vi "Set Output Values.vi"(8 "Error In":errorcluster, 9 "Start Index":i32, 10 "Values":dbl[](array[numeric]), 11 "BNT_ULx-MCSV in":refnum<class "BNT_ULx-MCSV.lvclass">) -> (0 "Error Out":errorcluster, 3 "BNT_ULx-MCSV out":refnum<class "BNT_ULx-MCSV.lvclass">)   [LabVIEW 2020, in "BNT_ULx.lvlib" / "BNT_ULx-MCSV.lvclass"]
doc: "Write voltage values to DAQmx device and publish.\n\nTimeout is set to constant 1s."
uses:
  BNT_ULx-MCSV.lvclass
  BNT_ULx-MCSV.lvclass/BNT_ULx-MCSV.ctl
  <vilib>/ULx/Write.llb/ULx Write (Analog 1D DBL NChan 1Samp).vi
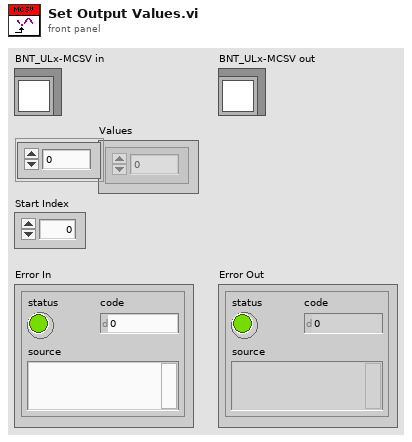
[diagram p1: front panel]
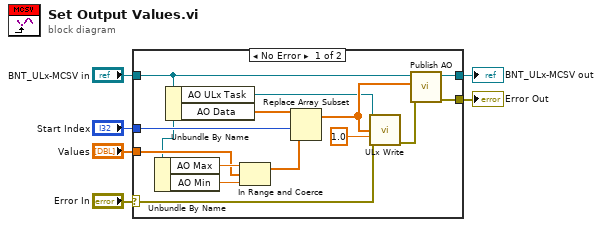
[diagram p0: block diagram]
diagram:
  n1 = case shown="No Error" "Error In" {
    selector: "Error In" -> [w10 w22]
    tunnel: [w12 w22] -> w5
    tunnel: [w13 w21] -> w3
    tunnel: "BNT_ULx-MCSV in" -> [w14 w21]
    tunnel: "Values" -> [w18 _]
    tunnel: "Start Index" -> [w15 _]
    frame No Error {
      n2 = Unbundle By Name(w14) -> ("AO Max"=w20:dbl, "AO Min"=w19:dbl)
      n3 = Unbundle By Name(w14) -> ("AO ULx Task"=w7:refnum<k24>, "AO Data"=w17:dbl[])
      n4 = In Range and Coerce(upper limit=w20, x=w18, lower limit=w19) -> (coerced(x)=w16:dbl[])  [unwired: 1 out]
      n5 = Replace Array Subset(array=w17, new element=w16, index=w15) -> (w8:dbl[])
      n6 = call-poly <vilib>:"ULx Write.vi"("task in"=w7, "data"=w8, "timeout"=1.0, "error in"=w10) -> ("error out"=w11:errorcluster)  [unwired: 9 in, 2 out]
      n7 = call "Publish AO.vi"("error in"=w11, "AO Data"=w8, "BNT_ULx-MCSV in"=w14) -> ("error out"=w12:errorcluster, "BNT_ULx-MCSV out"=w13:refnum<class "BNT_ULx-MCSV.lvclass">)  [unwired: 7 in]
    }
    frame Error {
    }
  }
  "Error Out" <- w5
  "BNT_ULx-MCSV out" <- w3
